vi "SA - wForms ABS MAX.vi"(0 "wForms IN":waveform(dbl)[](array[waveform])) -> (13 "ABS MAX's":dbl[](array[numeric]), 14 "wForms OUT":waveform(dbl)[](array[waveform]))   [LabVIEW 2020, in "GSwFormDSP.lvclass"]
uses:
  GSwFormDSP.lvclass
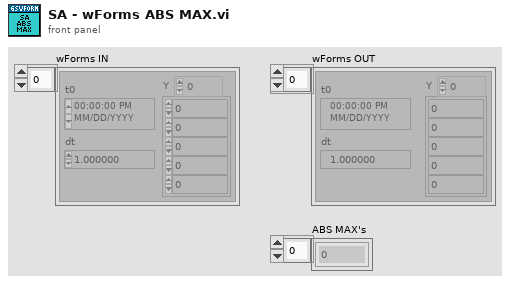
[diagram p1: front panel]
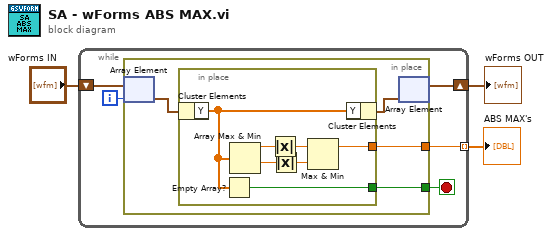
[diagram p0: block diagram]
diagram:
  n1 = while {
    shift-right: [w6] -> w2
    shift-left: "wForms IN" -> [w8]
    tunnel: [w5] -> w3 mode=indexing
    i -> [w7]
    stop <- w4 stop-if-true
    n2 = in-place {
      in-place-border: [w10] -> w5
      in-place-border: [w9] -> w4
      n3 = in-place-array #1(w8, w7) -> (w12:waveform(dbl))
      n4 = in-place {
        in-place-border: [w15] -> w10
        in-place-border: [w13] -> w9
        n5 = in-place-cluster #2(w12) -> ("Y"=w14:dbl[])
        n6 = Empty Array?(array=w14) -> (empty?=w13:bool)
        n7 = Array Max & Min(array=w14) -> (max value=w18:dbl, min value=w19:dbl)  [unwired: 2 out]
        n8 = Absolute Value(x=w18) -> (abs(x)=w17:dbl)
        n9 = Absolute Value(x=w19) -> (abs(x)=w16:dbl)
        n10 = Max & Min(x=w17, y=w16) -> (max(x,y)=w15:dbl)  [unwired: 1 out]
        n11 = in-place-cluster #2("Y"=w14) -> (w11:waveform(dbl))
      }
      n12 = in-place-array #1(w11) -> (w6:waveform(dbl)[])  [unwired: 1 out]
    }
  }
  "ABS MAX's" <- w3
  "wForms OUT" <- w2
